vi "abort Acquisition LV.vi"(8 "error in (no error)":errorcluster) -> (0 "error out":errorcluster)   [LabVIEW 2016, in "cameraLibrary.lvlib"]
doc: "Abort camera acquisition.\n\n\nvoid CAMERALIBRARYSHARED_EXPORT abortAcquisitionLV();"
uses:
  cameraLibrary.lvlib
  cameraLibrary.dll
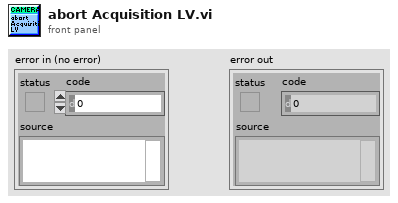
[diagram p1: front panel]
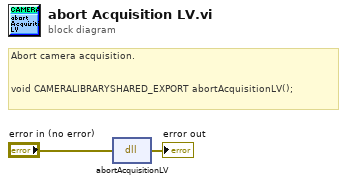
[diagram p0: block diagram]
diagram:
  # "Abort camera acquisition.\n\n\nvoid CAMERALIBRARYSHARED_EXPORT abortAcquisitionLV();"
  n1 = dll-call lib="C:/Users/TMM/repos/EXPRES/FEM/FTT/support/Camera Library/cameraLibrary.*" fn="abortAcquisitionLV"(error in="error in (no error)") -> (error out=→"error out":errorcluster)  [unwired: 3 in, 1 out]
